vi "Vision 2017.vi"() -> ()   [LabVIEW 2016]
uses:
  <vilib>/Rock Robotics/WPI/Camera/WPI_CameraImageSize.ctl
  Program Files (x86)/National Instruments/LabVIEW 2016/examples/FRC/roboRIO/Vision/2017 Vision Example/Vision Support Code/Camera Types.ctl
  <vilib>/Rock Robotics/WPI/Camera/WPI_CameraWhite Balance Values.ctl
  <vilib>/Rock Robotics/WPI/Camera/WPI_CameraExposure Values.ctl
  <vilib>/Rock Robotics/WPI/Camera/WPI_CameraFrameRate.ctl
  Robot Global Data.vi
  <vilib>/vision/NI_Vision_Development_Module.lvlib
panel:
  out "FOV ?":dbl
  in  "Camera Type":T1
  out "X":dbl
  in  "Std Devs for Calibration":cluster{"H":dbl, "S":dbl, "V":dbl}={"H"=4.0, "S"=6.0, "V"=6.0}
  in  "Image Size":T2=enum."320x240"
  out "Original Image":T3(plugin-control)
  out "Mask":T3(plugin-control)
  in  "LED Color":T4={"Hue"={48.52399131877658, 113.6727294921875}, "Sat"={34.78571428571429, 255.0}, "Val"={91.07142857142858, 255.0}} {"Hue" scale=0.0..255.0 scale format="%#_3g"}
  out "Qualified Particles":i32
  in  "Annotate":bool=TRUE
  out "Results":T5 {"Error" format="%#_3g"; "Pixels"."Rectangle"."Numeric 5" format="%#_3g"; "Pixels"."Rectangle"."Numeric 3" format="%#_3g"; "Pixels"."Rectangle"."Numeric 2" format="%#_3g"; "Pixels"."Rectangle"."Numeric" format="%#_3g"; "Normalized"."Rectangle"."Numeric 5" format="%#_2g"; "Normalized"."Rectangle"."Numeric 3" format="%#_2g"; "Normalized"."Rectangle"."Numeric 2" format="%#_2g"; "Normalized"."Rectangle"."Numeric" format="%#_2g"; "Normalized"."Center"."?" format="%#_3g"; "Normalized"."Center"."?" format="%#_3g"; "Distance (ft)" format="%#_3g"}
  in  "Score Cutoff":dbl=50.0
  in  "Particles":dbl=10.0
  in  "Color Mode":u16(ring)=3 items=["RGB", "HSL", "HSV", "HSI"]
  out "Top Score":dbl
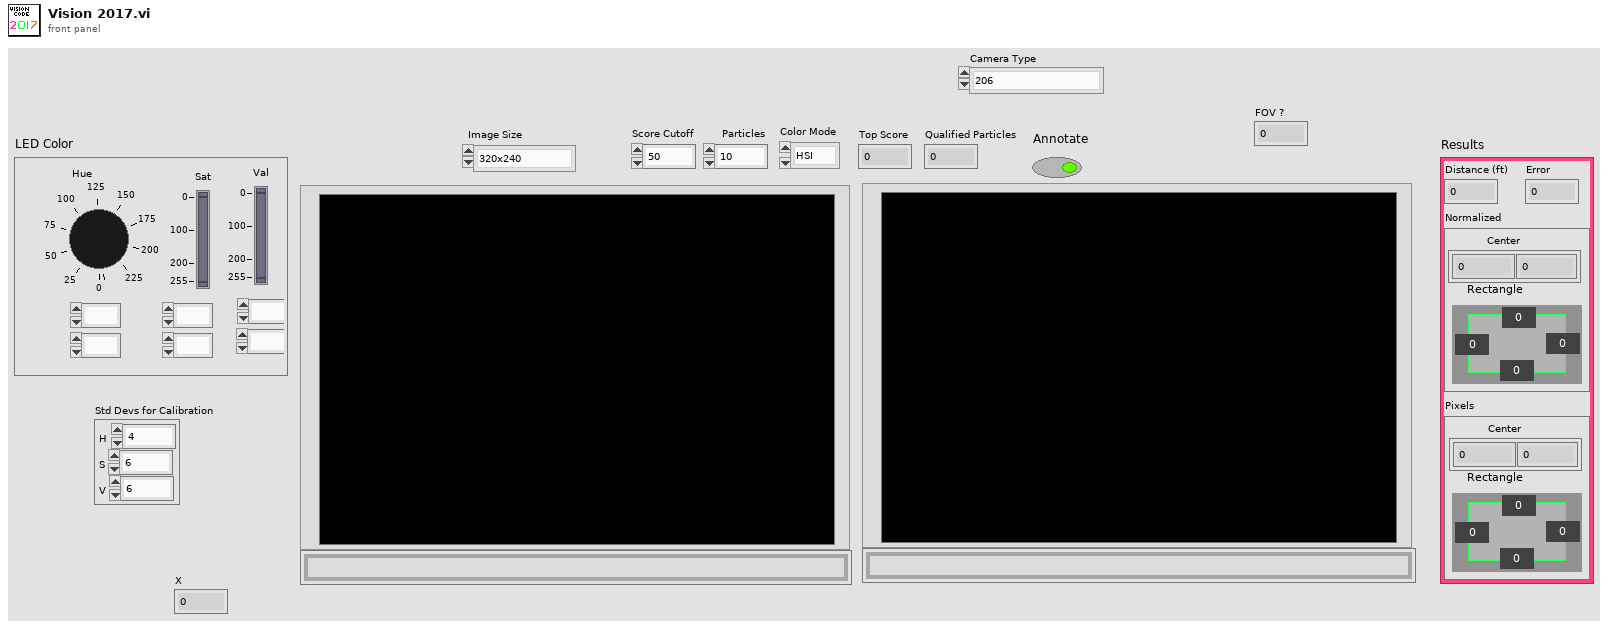
[diagram p1: front panel]
types:
  T1 = typedef "Camera Types.ctl" = enum16{"206", "1011", "1013", "MS HD3000 square", "MS HD3000 640x480"}
  T2 = typedef "WPI_CameraImageSize.ctl" = enum16{"640x480", "320x240", "160x120", "Custom"}
  T3 = typedef "IMAQ Image.ctl" = refnum<image>
  T4 = cluster{"Hue":cluster{dbl, dbl}, "Sat":cluster{dbl, dbl}, "Val":cluster{dbl, dbl}}
  T5 = cluster{"Distance (ft)":dbl, "Error":dbl, "Normalized":cluster{"Center":cluster{dbl, dbl}, "Rectangle":cluster{"Numeric":dbl, "Numeric 2":dbl, "Numeric 3":dbl, "Numeric 5":dbl}}, "Pixels":cluster{"Center":cluster{dbl, dbl}, "Rectangle":cluster{"Numeric":dbl, "Numeric 2":dbl, "Numeric 3":dbl, "Numeric 5":dbl}}}
  T6 = typedef "WPI_CameraFrameRate.ctl" = u32
  T7 = typedef "WPI_CameraExposure Values.ctl" = enum16{"Auto", "Flicker-free 50 Hz", "Flicker-free 60 Hz", "Hold current", "Custom"}
  T8 = typedef "WPI_CameraWhite Balance Values.ctl" = enum16{"Auto", "Fixed indoor", "Fixed outdoor 1", "Fixed outdoor 2", "Fixed fluorescent 1", "Fixed fluorescent 2", "Hold current", "Custom"}
  T9 = typedef "Particle Parameters" = i32
  T10 = typedef "Image Type" = u32
  T11 = typedef "WPI_CameraDevRef.ctl" = cluster{"Camera Address":string, "CameraStatus":errorcluster}
  T12 = cluster{cluster{dbl, dbl}, cluster{dbl, dbl}, cluster{dbl, dbl}}
  T13 = cluster{"Left":dbl, "Top":dbl, "Right":dbl, "Bottom":dbl}
  T14 = cluster{"Distance (ft)":dbl, "Score":dbl, "Normalized":cluster{"Center":cluster{dbl, dbl}, "Rectangle":cluster{"Numeric":dbl, "Numeric 2":dbl, "Numeric 3":dbl, "Numeric 5":dbl}}, "Pixels":cluster{"Center":cluster{dbl, dbl}, "Rectangle":cluster{"Numeric":dbl, "Numeric 2":dbl, "Numeric 3":dbl, "Numeric 5":dbl}}}
  T15 = cluster{"Center":cluster{dbl, dbl}, "Rectangle":cluster{"Numeric":dbl, "Numeric 2":dbl, "Numeric 3":dbl, "Numeric 5":dbl}}
  T16 = cluster{"Numeric":dbl, "Numeric 2":dbl, "Numeric 3":dbl, "Numeric 5":dbl}
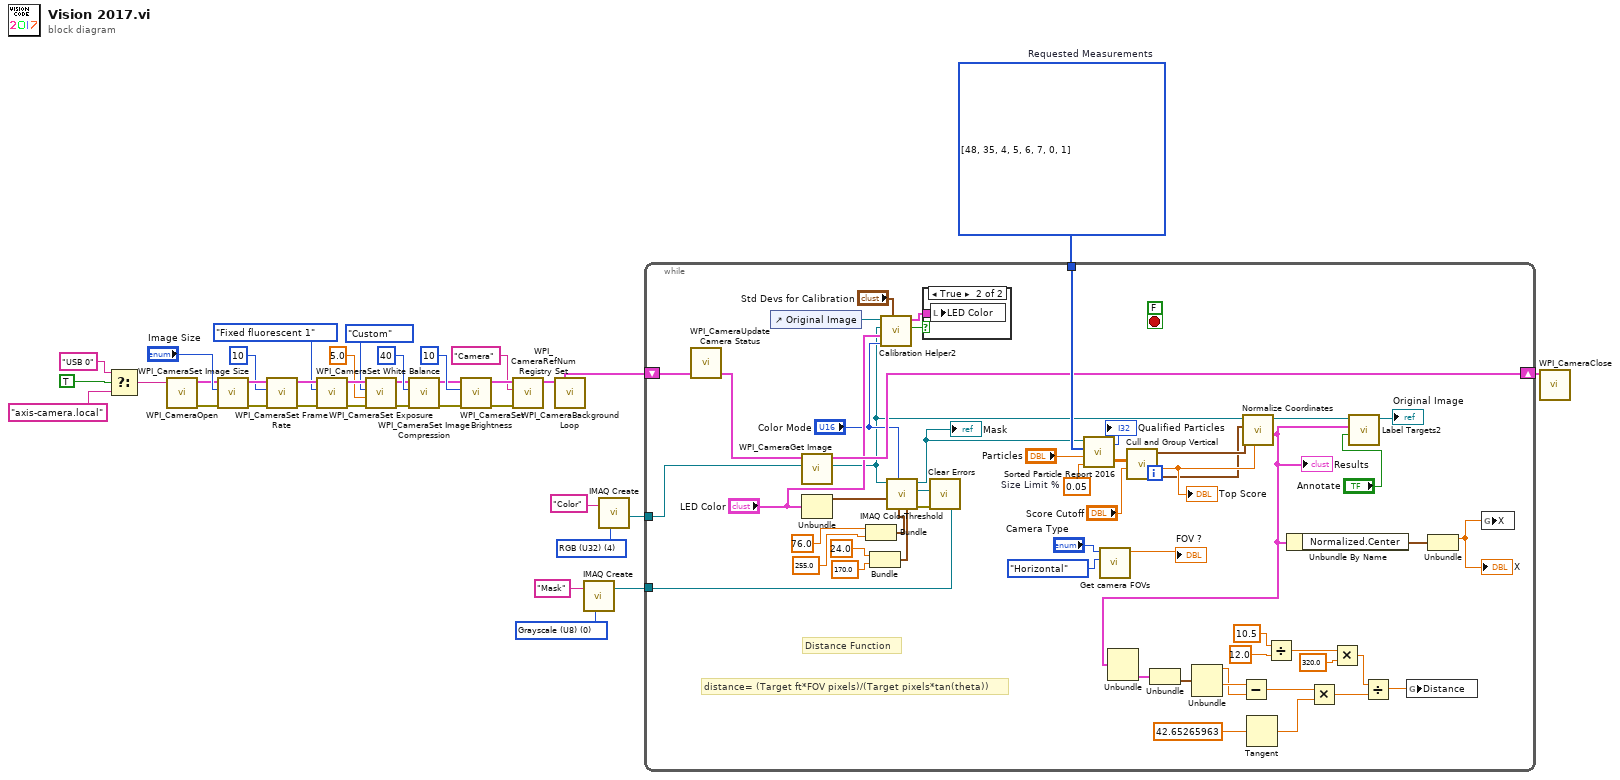
[diagram p0: block diagram]
diagram:
  w29 = T9[] [48, 35, 4, 5, 6, 7, 0, 1] items=["Center of Mass X", "Center of Mass Y", "First Pixel X", "First Pixel Y", "Bounding Rect Left", "Bounding Rect Top", "Bounding Rect Right", "Bounding Rect Bottom", "Max Feret Diameter Start X", "Max Feret Diameter Start Y", "Max Feret Diameter End X", "Max Feret Diameter End Y", "Max Horiz. Segment Length Left", "Max Horiz. Segment Length Right", "Max Horiz. Segment Length Row", "-", "Bounding Rect Width", "Bounding Rect Height", "Bounding Rect Diagonal", "Perimeter", "Convex Hull Perimeter", "Holes' Perimeter", "Max Feret Diameter", "Equivalent Ellipse Major Axis", "Equivalent Ellipse Minor Axis", "Equivalent Ellipse Minor Axis (Feret)", "Equivalent Rect Long Side", "Equivalent Rect Short Side", "Equivalent Rect Diagonal", "Equivalent Rect Short Side (Feret)", "Average Horiz. Segment Length", "Average Vert. Segment Length", "Hydraulic Radius", "Waddel Disk Diameter", "-", "Area", "Holes' Area", "Particle & Holes' Area", "Convex Hull Area", "Image Area", "-", "Number of Holes", "Number of Horiz. Segments", "Number of Vert. Segments", "-", "Orientation", "Max Feret Diameter Orientation", "-", "% Area/Image Area", "% Area/(Particle & Holes' Area)", "Ratio of Equivalent Ellipse Axes", "Ratio of Equivalent Rect Sides", "-", "Elongation Factor", "Compactness Factor", "Heywood Circularity Factor", "Type Factor", "-", "Sum X", "Sum Y", "Sum XX", "Sum XY", "Sum YY", "Sum XXX", "Sum XXY", "Sum XYY", "Sum YYY", "-", "Moment of Inertia XX", "Moment of Inertia XY", "Moment of Inertia YY", "Moment of Inertia XXX", "Moment of Inertia XXY", "Moment of Inertia XYY", "Moment of Inertia YYY", "Norm. Moment of Inertia XX", "Norm. Moment of Inertia XY", "Norm. Moment of Inertia YY", "Norm. Moment of Inertia XXX", "Norm. Moment of Inertia XXY", "Norm. Moment of Inertia XYY", "Norm. Moment of Inertia YYY", "Hu Moment 1", "Hu Moment 2", "Hu Moment 3", "Hu Moment 4", "Hu Moment 5", "Hu Moment 6", "Hu Moment 7"]  # Requested Measurements
  w32 = T10 0 items=["Grayscale (U8)", "Grayscale (I16)", "Grayscale (SGL)", "Complex (CSG)", "RGB (U32)", "HSL (U32)", "RGB (U64)", "Grayscale (U16)"] ("Image Type")
  w34 = T10 4 items=["Grayscale (U8)", "Grayscale (I16)", "Grayscale (SGL)", "Complex (CSG)", "RGB (U32)", "HSL (U32)", "RGB (U64)", "Grayscale (U16)"] ("Image Type")
  n1 = Select(t="USB 0" ("format string"), s=TRUE ("dot notation? (F)"), f="axis-camera.local" ("format string")) -> (s? t:f=w4:string)
  n2 = call <vilib>:"WPI_CameraOpen.vi"("Camera Address"=w4) -> ("error out"=w16:errorcluster, "CameraDevRef"=w17:T11)  [unwired: 1 in, 8 out]
  n3 = call <vilib>:"WPI_CameraSet Image Size.vi"("error in (no error)"=w16, "Image Size"="Image Size", "CameraDevRef"=w17) -> ("error out"=w15:errorcluster, "CameraDevRef Out"=w18:T11)  [unwired: 1 in, 6 out]
  n4 = call <vilib>:"WPI_CameraSet Frame Rate.vi"("error in (no error)"=w15, "Frame Rate (fps)"=T6 10, "CameraDevRef"=w18) -> ("error out"=w14:errorcluster, "CameraDevRef Out"=w20:T11)  [unwired: 7 out]
  n5 = call <vilib>:"WPI_CameraSet White Balance.vi"("error in (no error)"=w14, "White Balance"=WPI_CameraWhite_Balance_Values."Fixed fluorescent 1", "CameraDevRef"=w20) -> ("error out"=w13:errorcluster, "CameraDevRef Out"=w19:T11)  [unwired: 1 in, 6 out]
  n6 = call <vilib>:"WPI_CameraSet Exposure.vi"("error in (no error)"=w13, "Exposure (%)"=5.0, "Exposure"=WPI_CameraExposure_Values."Custom", "CameraDevRef"=w19) -> ("error out"=w12:errorcluster, "CameraDevRef Out"=w22:T11)  [unwired: 6 out]
  n7 = call <vilib>:"WPI_CameraSet Image Compression.vi"("error in (no error)"=w12, "Compression"=40, "CameraDevRef"=w22) -> ("error out"=w11:errorcluster, "CameraDevRef Out"=w21:T11)  [unwired: 7 out]
  n8 = call <vilib>:"WPI_CameraSet Brightness.vi"("error in (no error)"=w11, "Brightness"=10, "CameraDevRef"=w21) -> ("error out"=w10:errorcluster, "CameraDevRef Out"=w28:T11)  [unwired: 7 out]
  n9 = call <vilib>:"WPI_CameraRefNum Registry Set.vi"("error in (no error)"=w10, "refnum name"="Camera", "CameraDevRef"=w28) -> ("CameraDevRef"=w2:T11)  [unwired: 1 in, 7 out]
  n10 = call <vilib>:"WPI_CameraBackground Loop.vi"("CameraDevRef"=w2) -> ()  [unwired: 11 in]
  n11 = call "IMAQ Create"("Image Name"="Mask", "Image Type"=w32) -> ("New Image"=w30:T3)  [unwired: 2 in, 2 out]
  n12 = call "IMAQ Create"("Image Name"="Color", "Image Type"=w34) -> ("New Image"=w33:T3)  [unwired: 2 in, 2 out]
  n13 = while {
    tunnel: w33 -> [w72]
    tunnel: w30 -> [w88]
    tunnel: w29 -> [w86]
    shift-right: [w71] -> w1
    shift-left: w2 -> [w73]
    stop <- FALSE stop-if-true
    w84 = 0.05  # Size Limit %
    # "distance= (Target ft*FOV pixels)/(Target pixels*tan(theta))"
    # "Distance Function"
    n14 = call <vilib>:"WPI_CameraUpdate Camera Status.vi"("CameraDevRef In"=w73) -> ("CameraDevRef Out"=w74:T11)  [unwired: 4 in]
    n15 = control-ref of="Original Image"() -> (w65:refnum<vi>)
    n16 = call <vilib>:"WPI_CameraGet Image.vi"("Image"=w72, "CameraDevRef"=w74) -> ("Image Out"=w63:T3, "CameraDevRef Out"=w71:T11)  [unwired: 7 in, 1 out]
    n17 = Unbundle("LED Color") -> ("Hue"=w87:cluster{dbl, dbl})  [unwired: 2 out]
    n18 = Bundle(76.0, 255.0) -> (w51:cluster{dbl, dbl})  [unwired: 1 in]
    n19 = Bundle(24.0, 170.0) -> (w54:cluster{dbl, dbl})  [unwired: 1 in]
    n20 = call "Calibration Helper2.vi"("Std Devs"="Std Devs for Calibration", "Color Mode"="Color Mode", "Color Components"="LED Color", "Image"=w63, "Image Ctl Refnum"=w65) -> ("Changed"=w67:bool, "output color"=w66:T12)  [unwired: 5 in]
    n21 = call "IMAQ ColorThreshold"("Blue or Luma or Val or Inten Range"=w54, "Green or Sat Range"=w51, "Color Mode"="Color Mode", "Red or Hue Range"=w87, "Image Dst"=w88, "Image Src"=w63) -> ("error out"=w82:errorcluster, "Image Dst Out"=w79:T3)  [unwired: 4 in]
    "Mask" <- w79
    n22 = case shown="True" w67 {
      tunnel: w66 -> [_ w90]
      frame False {
      }
      frame True {
        n23 = local write "LED Color"(w90) -> ()
      }
    }
    n24 = call <vilib>:"Clear Errors.vi"("error in (no error)"=w82) -> ()  [unwired: 5 in, 2 out]
    n25 = call "Sorted Particle Report 2016.vi"("Min Area Size %"=w84, "Particle Count Limit"="Particles", "Pixel Measurements"=w86, "Image in"=w79) -> ("Sorted Data"=w81:dbl[][], "Particles"=→"Qualified Particles":i32)
    n26 = call "Get camera FOVs.vi"("Type"=enum16{"Horizontal", "Vertical", "Diagonal"}."Horizontal" ("Angle"), "Camera Type"="Camera Type") -> ("FOV"=→"FOV ?":dbl)  [unwired: 8 in, 1 out]
    n27 = call "Cull and Group Vertical.vi"("Score Cutoff"="Score Cutoff", "Sorted Data"=w81) -> ("Rect"=w64:T13, "Top Score"=w75:dbl, "Center"=w77:cluster{"X":dbl, "Y":dbl})  [unwired: 7 in]
    "Top Score" <- w75
    n28 = call "Normalize Coordinates.vi"("Score"=w75, "Center"=w77, "Bounding box"=w64, "Image in"=w63) -> ("Results"=w50:T14, "Image out"=w78:T3)  [unwired: 6 in]
    "Results" <- w50
    n29 = Unbundle(w50) -> ("Pixels"=w49:T15)  [unwired: 3 out]
    n30 = Unbundle(w49) -> ("Rectangle"=w48:T16)  [unwired: 1 out]
    n31 = Unbundle(w48) -> ("Numeric"=w45:dbl, "Numeric 3"=w46:dbl)  [unwired: 2 out]
    n32 = Subtract(x=w46, y=w45) -> (x-y=w44:dbl)
    n33 = Tangent(1:42.65265963) -> (0:w43:dbl)
    n34 = Divide(x=10.5, y=12.0) -> (x/y=w39:dbl)
    n35 = Unbundle By Name(w50) -> ("Normalized.Center"=w60:cluster{dbl, dbl})
    n36 = Multiply(x=w44, y=w43) -> (x*y=w38:dbl)
    n37 = Multiply(x=w39, y=320.0) -> (x*y=w37:dbl)
    n38 = call "Label Targets2.vi"("Annotate"="Annotate", "Results"=w50, "Image in"=w78) -> ("Image out"=→"Original Image":T3)  [unwired: 8 in]
    n39 = Divide(x=w37, y=w38) -> (x/y=w36:dbl)
    n40 = global write "Robot Global Data.vi" "Distance"(w36) -> ()
    n41 = Unbundle(w60) -> (w58:dbl)  [unwired: 1 out]
    "X" <- w58
    n42 = global write "Robot Global Data.vi" "X"(w58) -> ()
  }
  n43 = call <vilib>:"WPI_CameraClose.vi"("CameraDevRef"=w1) -> ()  [unwired: 1 in, 10 out]
